vi "Script Msg VI.vi"(6 "Name":string, 8 "error in":errorcluster, 9 "Ref.Msg VI":refnum<vi>, 10 "Conpane Map":T1(c390)) -> (0 "error out":errorcluster)   [LabVIEW 2025, in "_Msg Rescript.lvlib" / "_Msg Rescript.lvclass"]
uses:
  _Msg Rescript.lvclass
  _Msg Rescript.lvclass/_Msg Rescript.ctl
  <vilib>/Utility/traverseref.llb/TRef TravTarget.ctl
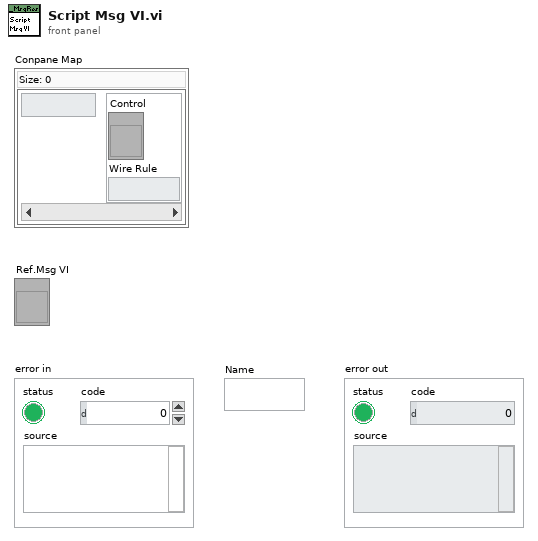
[diagram p1: front panel]
types:
  T1 = map{i32, cluster{"Control":refnum<vi>, "Wire Rule":enum16{"Invalid Wire Rule", "Required", "Recommended", "Optional", "Dynamic Dispatch"}}}
  T2 = typedef "TRef TravTarget.ctl" = enum16{"FP", "BD", "Other"}
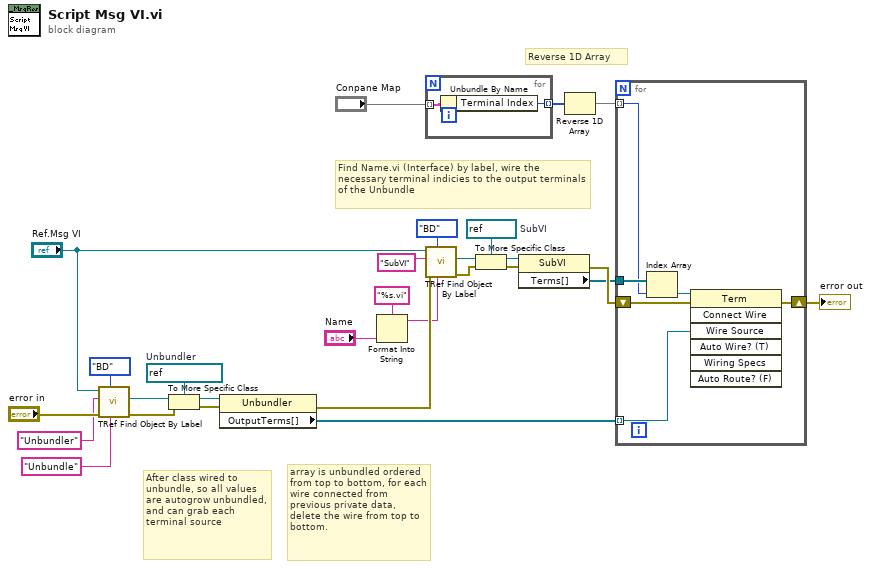
[diagram p0: block diagram]
diagram:
  w10 = refnum<vi> refnum  # Unbundler
  w27 = refnum<vi> refnum  # SubVI
  # "Reverse 1D Array"
  # "array is unbundled ordered from top to bottom, for each wire connected from previous private data, delete the wire from top to bottom."
  # "After class wired to unbundle, so all values are autogrow unbundled, and can grab each terminal source"
  # "Find Name.vi (Interface) by label, wire the necessary terminal indicies to the output terminals of the Unbundle"
  n1 = call <vilib>:"TRef Find Object By Label.vi"("Label"="Unbundle", "Traverse Target"=TRef_TravTarget."BD", "error in (no error)"="error in", "Class Name"="Unbundler", "VI Ref"="Ref.Msg VI") -> ("error out"=w11:errorcluster, "Found Obj Ref"=w9:refnum<vi>)  [unwired: 3 in, 2 out]
  n2 = To More Specific Class(target class=w10, reference=w9, error in=w11) -> (specific class reference=w6:refnum<vi>, error out=w2:errorcluster)
  n3 = property class="Unbundler"(reference=w6, error in=w2) -> (error out=w17:errorcluster, "OutputTerms[]"=w1:refnum<vi>[])  [unwired: 1 out]
  n4 = Format Into String(format string="%s.vi", "Name") -> (resulting string=w12:string)  [unwired: 2 in, 1 out]
  n5 = for {
    tunnel: "Conpane Map" -> [w30] mode=indexing
    tunnel: [w29] -> w22 mode=indexing
    n6 = Unbundle By Name(w30) -> ("Terminal Index"=w29:i32)
  }
  n7 = call <vilib>:"TRef Find Object By Label.vi"("Label"=w12, "Traverse Target"=TRef_TravTarget."BD", "error in (no error)"=w17, "Class Name"="SubVI", "VI Ref"="Ref.Msg VI") -> ("error out"=w26:errorcluster, "Found Obj Ref"=w16:refnum<vi>)  [unwired: 3 in, 2 out]
  n8 = To More Specific Class(target class=w27, reference=w16, error in=w26) -> (specific class reference=w24:refnum<vi>, error out=w23:errorcluster)
  n9 = property class="SubVI"(reference=w24, error in=w23) -> (error out=w21:errorcluster, "Terms[]"=w20:refnum<vi>[])  [unwired: 1 out]
  n10 = Reverse 1D Array(array=w22) -> (reversed array=w18:i32[])
  n11 = for {
    tunnel: w20 -> [w36]
    tunnel: w18 -> [w35] mode=indexing
    shift-right: [w32] -> w13
    shift-left: w21 -> [w33]
    tunnel: w1 -> [w31] mode=indexing
    n12 = Index Array(array=w36, index=w35) -> (element=w34:refnum<vi>)
    n13 = invoke class="Term" method="Connect Wire"(reference=w34, error in=w33, "Wire Source"=w31) -> (error out=w32:errorcluster)  [unwired: 4 in, 6 out]
  }
  "error out" <- w13
